vi "Axis modifications.vi"(1 "Driver JoyStick Info":cluster{"Slow Drive?":bool, "Axisses":dbl[]}) -> (0 "Driver JoyStick Info Out":cluster{"Slow Drive?":bool, "Axisses":dbl[]})   [LabVIEW 2012]
uses:
  Drive Global Data.vi
panel:
  # "Out"
  # "In"
  # "X"
  # "Y"
  # "X"
  # "Y"
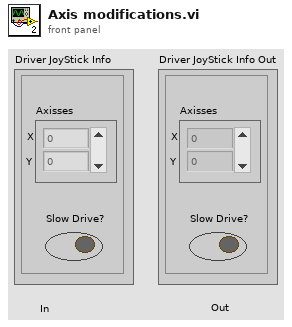
[diagram p1: front panel]
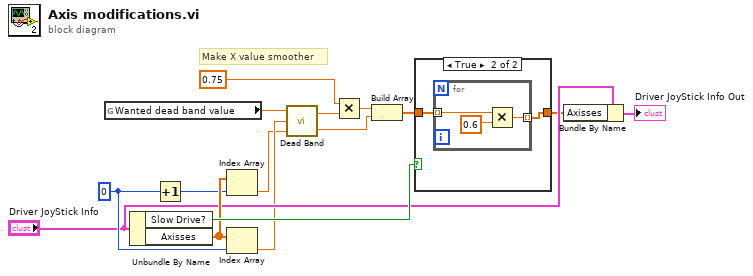
[diagram p0: block diagram]
diagram:
  w12 = 0 ("index")
  # "Make X value smoother"
  n1 = global read "Drive Global Data.vi" "Wanted dead band value"() -> (w1:dbl)
  n2 = Unbundle By Name("Driver JoyStick Info") -> ("Slow Drive?"=w15:bool, "Axisses"=w14:dbl[])
  n3 = Increment(x=w12) -> (x+1=w13:i32)
  n4 = Index Array(array=w14, index=w13) -> (element=w4:dbl)
  n5 = Index Array(array=w14, index=w12) -> (element=w5:dbl)
  n6 = call "Dead Band.vi"("Axis 2 In"=w4, "Axis 1 In"=w5, "Dead Band"=w1) -> ("Axis 2 Out"=w2:dbl, "Axis 1 Out"=w3:dbl)
  n7 = Multiply(x=0.75, y=w3) -> (x*y=w6:dbl)
  n8 = Build Array(w6, w2) -> (w8:dbl[])
  n9 = case shown="True" w15 {
    tunnel: [w16 w17] -> w7
    tunnel: w8 -> [w16 w18]
    frame False {
    }
    frame True {
      n10 = for {
        tunnel: w18 -> [w21] mode=indexing
        tunnel: [w19] -> w17 mode=indexing
        n11 = Multiply(x=w21, y=0.6) -> (x*y=w19:dbl)
      }
    }
  }
  n12 = Bundle By Name(cluster="Driver JoyStick Info", "Axisses"=w7) -> (→"Driver JoyStick Info Out":cluster{"Slow Drive?":bool, "Axisses":dbl[]})
